vi "cel to far.vi"() -> ()   [LabVIEW 2009]
panel:
  out "Thermometer 2":dbl(slide) scale=0.0..100.0
  out "fareh":dbl
  in  "celcius":dbl
  out "Thermometer":dbl(slide) scale=0.0..100.0
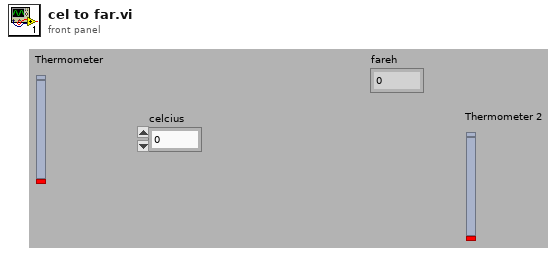
[diagram p1: front panel]
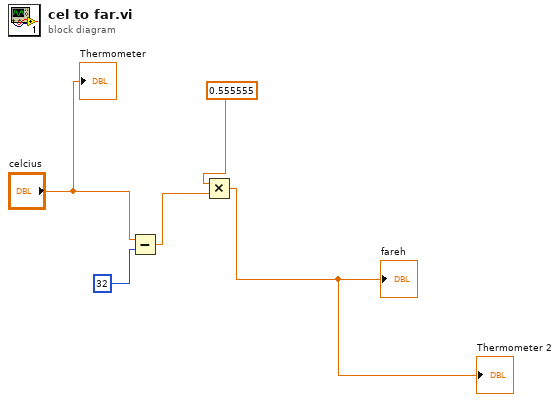
[diagram p0: block diagram]
diagram:
  n1 = Subtract(x="celcius", y=32) -> (x-y=w5:dbl)
  n2 = Multiply(x=0.555555, y=w5) -> (x*y=→"fareh" →"Thermometer 2":dbl)
  "Thermometer" <- "celcius"
